vi "FTP_PASS.vi"(0 "connection ID":refnum<k5>, 1 "password":string, 2 "error in":errorcluster) -> (3 "connection ID out":refnum<k5>, 4 "reply string":string, 5 "Good Reply?":bool, 6 "error out":errorcluster)   [LabVIEW 2012]
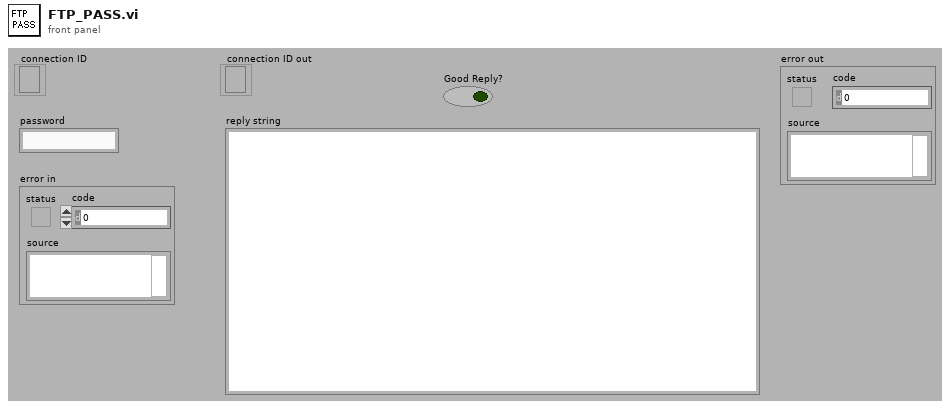
[diagram p1: front panel]
types:
  T1 = enum16{"unknown", "100 + Prelim", "200 + ", "300 + Intermed", "400 - Transient", "500 - Permanent"}
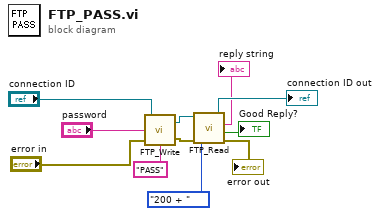
[diagram p0: block diagram]
diagram:
  n1 = call <userlib>:"FTP_Write.vi"("Cmd"="PASS", "error in"="error in", "data"="password", "connection ID in"="connection ID") -> ("error out"=w2:errorcluster, "connection ID out"=w3:refnum<k5>)
  n2 = call <userlib>:"FTP_Read.vi"("error In"=w2, "expected class"=T1."200 + ", "connection ID"=w3) -> ("error out"=→"error out":errorcluster, "Good Reply?"=→"Good Reply?":bool, "reply string"=→"reply string":string, "connection ID out"=→"connection ID out":refnum<k5>)  [unwired: 1 out]
